vi "getValueAsU8.vi"(8 "error in (no error)":errorcluster, 11 "type.U8 in":refnum<class "type.U8.lvclass">) -> (0 "error out":errorcluster, 2 "value":u8, 3 "type.U8 out":refnum<class "type.U8.lvclass">)   [LabVIEW 2013, in "type.U8.lvclass"]
uses:
  type.U8.lvclass
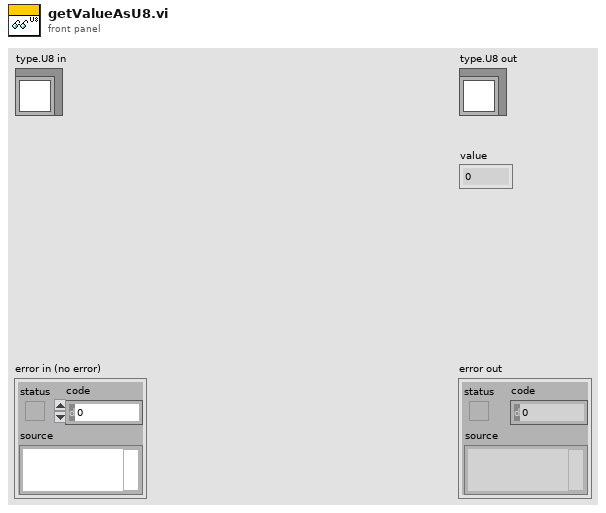
[diagram p1: front panel]
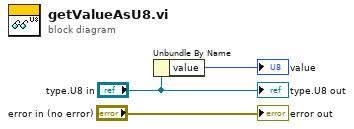
[diagram p0: block diagram]
diagram:
  n1 = Unbundle By Name("type.U8 in") -> ("value"=→"value":u8)
  "error out" <- "error in (no error)"
  "type.U8 out" <- "type.U8 in"
